vi "FLiBe Density.vi"(11 "Pri Temp (K)":dbl) -> (3 "Primary Density (kg/m^3)":dbl)   [LabVIEW 2019]
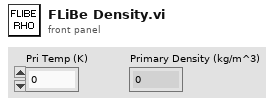
[diagram p1: front panel]
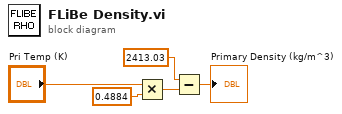
[diagram p0: block diagram]
diagram:
  n1 = Multiply(x="Pri Temp (K)", y=0.4884) -> (x*y=w4:dbl)
  n2 = Subtract(x=2413.03, y=w4) -> (x-y=→"Primary Density (kg/m^3)":dbl)
